vi "Write SSM Value.vi"(8 "error in":errorcluster, 10 "SSM value":u8 format="%02b", 11 "32-bit Word in":refnum<class "32-bit Word.lvclass">) -> (0 "error out":errorcluster, 3 "32-bit Word out":refnum<class "32-bit Word.lvclass">)   [LabVIEW 2020, in "32-bit Word.lvclass"]
uses:
  32-bit Word.lvclass
  32-bit Word.lvclass/32-bit Word.ctl
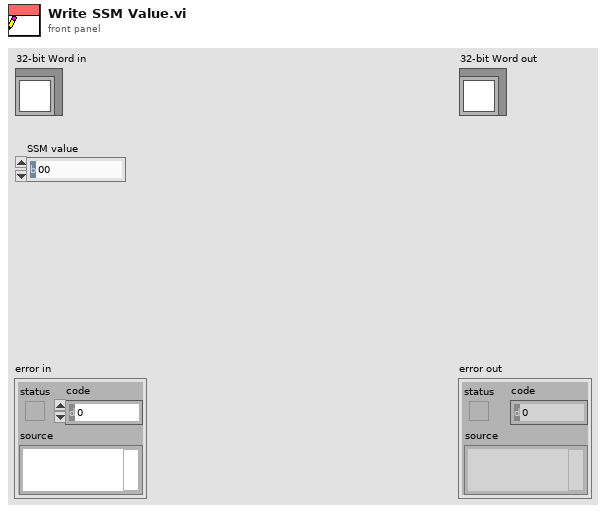
[diagram p1: front panel]
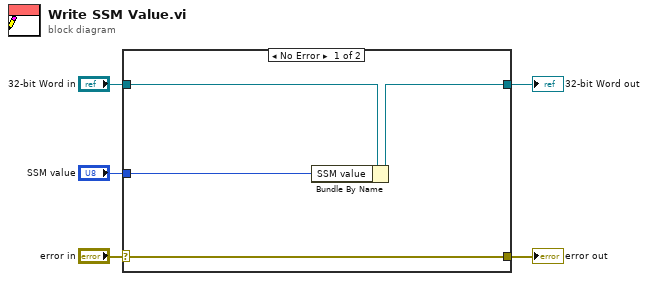
[diagram p0: block diagram]
diagram:
  n1 = case shown="No Error" "error in" {
    selector: "error in" -> [w9 w10]
    tunnel: [w9 w10] -> w4
    tunnel: [w7 w11] -> w2
    tunnel: "32-bit Word in" -> [w8 w11]
    tunnel: "SSM value" -> [w6 _]
    frame No Error {
      n2 = Bundle By Name(cluster=w8, "SSM value"=w6) -> (w7:refnum<class "32-bit Word.lvclass">)
    }
    frame Error {
    }
  }
  "error out" <- w4
  "32-bit Word out" <- w2
